vi "XML Script - Attribute String.vi"(1 "Attribute String":string, 2 "XML Script Attribute":T1) -> (0 "XML Script - Attribute String":string)   [LabVIEW 2017]
uses:
  <vilib>/_script/XML Scripting/XML Script Attribute.ctl
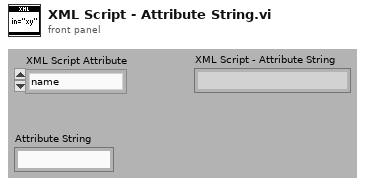
[diagram p1: front panel]
types:
  T1 = typedef "XML Script Attribute.ctl" = enum16{"name", "style", "path", "position", "in", "out", "width", "height", "index", "value", "default", "location", "offset", "typeindex", "size", "source", "destination", "indicator", "type", "controlname", "label", "conpaneidx", "mode", "description", "hasCondTerm", "linkIdentity", "caseselectortype", "concatInputs", "inName", "instantiationpath", "loopCondition", "IndexMode", "formulaInputs", "formulaOutputs", "msnFuncName", "msnIsDynamic", "msnIsODEUserFunction", "ignoreSearchDialog"}
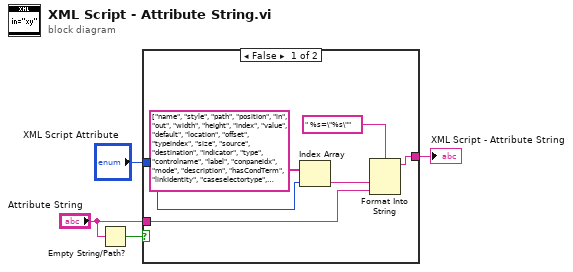
[diagram p0: block diagram]
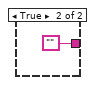
[diagram p2: hidden frame]
diagram:
  n1 = Empty String/Path?(string/path="Attribute String") -> (empty?=w3:bool)
  n2 = case shown="False" w3 {
    tunnel: [w6 ""] -> w1
    tunnel: "XML Script Attribute" -> [w9 _]
    tunnel: "Attribute String" -> [w7 _]
    frame False {
      n3 = Index Array(array=string[] ["name", "style", "path", "position", "in", "out", "width", "height", "index", "value", "default", "location", "offset", "typeindex", "size", "source", "destination", "indicator", "type", "controlname", "label", "conpaneidx", "mode", "description", "hasCondTerm", "linkIdentity", "caseselectortype", "concatInputs", "inName", "instantiationpath", "loopCondition", "IndexMode", "formulaInputs", "formulaOutputs", "msnFuncName", "msnIsDynamic", "msnIsODEUserFunction", "IgnoreSearchDialog"] ("Strings []"), index=w9) -> (element=w8:string)
      n4 = Format Into String(format string=" %s=\"%s\"", w8, w7) -> (resulting string=w6:string)  [unwired: 2 in, 1 out]
    }
    frame True {
    }
  }
  "XML Script - Attribute String" <- w1
